vi "Set base-path.vi"(8 "error in (no error)":errorcluster, 10 "base-path":string, 11 "URI-Component.Path in":refnum<class "URI-Component.Path.lvclass">) -> (0 "error out":errorcluster, 3 "URI-Component.Path out":refnum<class "URI-Component.Path.lvclass">)   [LabVIEW 2013, in "openURI.lvlib" / "URI-Component.Path.lvclass"]
uses:
  URI-Component.Path.lvclass
  URI-Component.Path.lvclass/URI-Component.Path.ctl
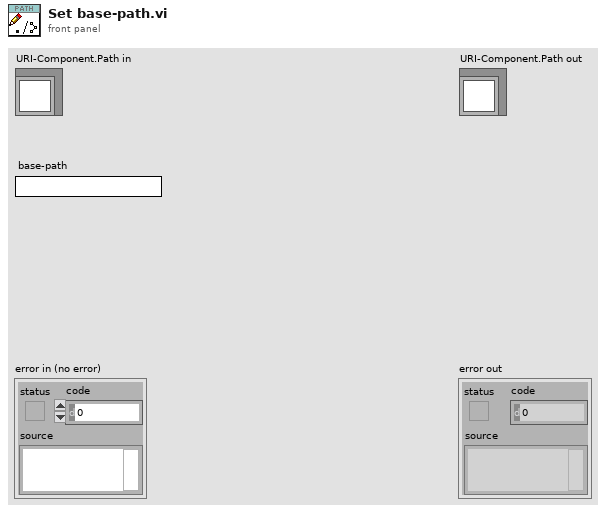
[diagram p1: front panel]
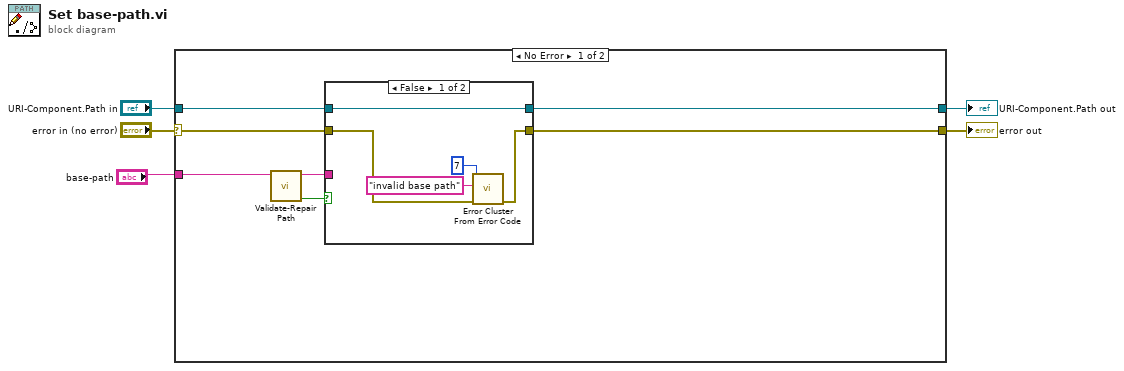
[diagram p0: block diagram]
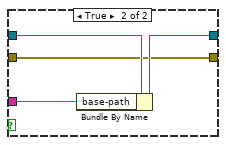
[diagram p2: hidden frame]
diagram:
  n1 = case shown="No Error" "error in (no error)" {
    selector: "error in (no error)" -> [w7 w23]
    tunnel: [w6 w23] -> w4
    tunnel: [w11 w22] -> w2
    tunnel: "URI-Component.Path in" -> [w12 w22]
    tunnel: "base-path" -> [w10 _]
    frame No Error {
      n2 = call "Validate-Repair Path.vi"("path in"=w10) -> ("Valid"=w8:bool, "path out"=w9:string)  [unwired: 7 in, 2 out]
      n3 = case shown="False" w8 {
        tunnel: w12 -> [w17 w21]
        tunnel: [w17 w20] -> w11
        tunnel: w9 -> [_ w19]
        tunnel: w7 -> [w15 w18]
        tunnel: [w16 w18] -> w6
        frame False {
          n4 = call <vilib>:"Error Cluster From Error Code.vi"("error in (no error)"=w15, "error message (\"\")"="invalid base path" ("error message (\"\")"), "error code (0)"=7) -> ("error out"=w16:errorcluster)  [unwired: 6 in]
        }
        frame True {
          n5 = Bundle By Name(cluster=w21, "base-path"=w19) -> (w20:refnum<class "URI-Component.Path.lvclass">)
        }
      }
    }
    frame Error {
    }
  }
  "error out" <- w4
  "URI-Component.Path out" <- w2
